vi "Main.vi"() -> ()   [LabVIEW 2017, in "MQTT.lvlib"]
doc: "This template is based from the Queued Message Handler design pattern and the Queued Message Handler Project Template that ships with LabVIEW 2014.\n\nThe main difference is that the Queue is private to this module and communication between modules is done via Broadcast and Requests events.\n\nRequests events are wrapped via public API methods and are handled in the Event handler loop in this VI.\nAny module can register for Broadcast events sent by this module.\n\nThe Event Handling Loop generates messages based on user interface actions.\n\nThe Message Handling Loop processes messages generated by the Event Handling Loop, or by other messages. The messages are string values, so new messages can be added easily to the Message Cases case structure in the Message Handling Loop. Each message cluster can also provide an optional value for Message Data, which is a variant that can be converted to whatever message-specific data is required.\n_____\nBased on Delacor QMH Project Template 3.1.0.34."
uses:
  MQTT.lvlib
  <vilib>/Delacor/Delacor QMH/Libraries/Cloneable Module Admin_class/Delacor_lib_QMH_Cloneable Module Admin.lvclass
  C:/Program Files (x86)/National Instruments/LabVIEW 2017/vi.lib/Delacor/Delacor QMH/Libraries/Module Admin_class/Delacor_lib_QMH_Module Admin.lvclass
  MessageTypedef.ctl
  Module Data--cluster.ctl
  OOP/MQTTclient.lvclass
  OOP/Dict/DICT.lvclass
  <vilib>/Delacor/Delacor QMH/Libraries/Message Queue_class/Delacor_lib_QMH_Message Queue.lvclass/Delacor_lib_QMH_Message Queue.ctl
  <vilib>/Delacor/Delacor QMH/Libraries/Cloneable Module Admin_class/Delacor_lib_QMH_Cloneable Module Admin.lvclass/Delacor_lib_QMH_Cloneable Module Admin.ctl
  Stop Argument--cluster.ctl
  <vilib>/Delacor/Delacor QMH/Libraries/Module Admin_class/Delacor_lib_QMH_Module Admin.lvclass/Delacor_lib_QMH_Module Admin.ctl
  Configure Argument--cluster.ctl
  Connect Argument--cluster.ctl
  disconnect Argument--cluster.ctl
  Subscrie Argument--cluster.ctl
  unsubscribe Argument--cluster.ctl
  Publish Argument--cluster.ctl
  broadcastTopic Argument--cluster.ctl
  PublishByAlias Argument--cluster.ctl
  addTopicAlias Argument--cluster.ctl
  <vilib>/Utility/miscctls.llb/LVPointTypeDef.ctl
  OOP/MQTT1/MQTT1.lvclass
  C:/Users/radzi01m/OneDrive - SIEMENSGAMESA/ISYS/MQTTGateway/OOP/MQTTclient.lvclass
  <vilib>/Delacor/Delacor QMH/Libraries/Message Queue_class/Delacor_lib_QMH_Enqueue Message (Single).vi
  <vilib>/Delacor/Delacor QMH/Libraries/Cloneable Module Admin_class/Delacor_lib_QMH_Get Module ID.vi
  <vilib>/Delacor/Delacor QMH/Libraries/Module Admin_class/Delacor_lib_QMH_Get External Launch.vi
  <vilib>/Utility/error.llb/Error Cluster From Error Code.vi
  <vilib>/ErrorRing/Error Ring.xnode
  <vilib>/Delacor/Delacor QMH/Libraries/Message Queue_class/Delacor_lib_QMH_Message Queue.lvclass
  Clone Registration/Clone Registration.lvlib
panel:
  in  "Simulate MHL Error":bool
  in  "Simulate EHL Error":bool
  out "error out":errorcluster
  in  "Module Admin":refnum<class "Delacor_lib_QMH_Cloneable Module Admin.lvclass">
  out "Status":string
  # "Other QMH Modules communicate with this Module via its Public API (wrappers for its Request Events).\n\nThis Module communicates with other Modules via its Broadcast Events.\nAny module that wants to get these messages, just registers for this module's Broadcast events."
  # "This template is for the Delacor Modified Queued Message Handler design pattern.\n\nSee the block diagram for more information on how to use this template."
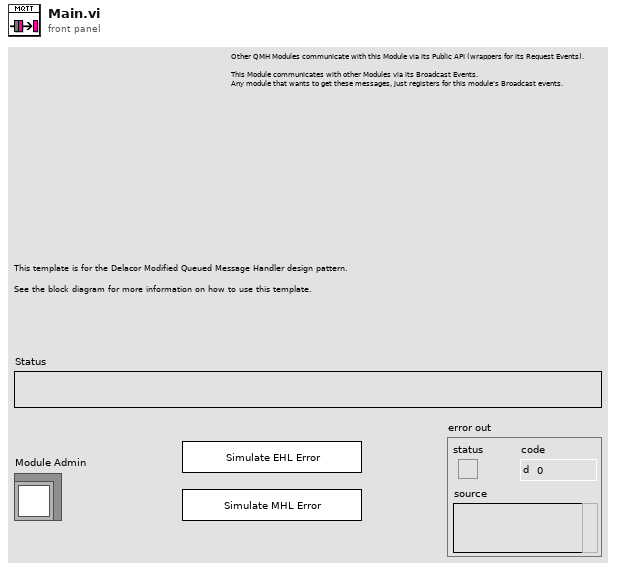
[diagram p1: front panel]
types:
  T1 = typedef "MQTT.lvlib/Request Events--cluster.ctl" = cluster{"Stop Module":refnum<user-event>, "Show Panel":refnum<user-event>, "Hide Panel":refnum<user-event>, "Show Diagram":refnum<user-event>, "Get Module Execution Status":refnum<user-event>, "Configure":refnum<user-event>, "Connect":refnum<user-event>, "disconnect":refnum<user-event>, "Subscrie":refnum<user-event>, "unsubscribe":refnum<user-event>, "Publish":refnum<user-event>, "Register Event":refnum<user-event>, "broadcastTopic":refnum<user-event>, "PublishByAlias":refnum<user-event>, "addTopicAlias":refnum<user-event>}
  T2 = typedef "MQTT.lvlib/Module Data--cluster.ctl" = cluster{"Status":string, "MQTTclient":refnum<class "MQTTclient.lvclass">, "DICT":refnum<class "DICT.lvclass">}
  T3 = typedef "MQTT.lvlib/Stop Argument--cluster.ctl" = cluster{"Origin":string, "Module ID":i32, "Exit via Stop Module Req?":bool, "Wait for Module to stop?":bool}
  T4 = typedef "MQTT.lvlib/Configure Argument--cluster.ctl" = cluster{"Module ID":i32, "JSON config":string}
  T5 = typedef "MQTT.lvlib/Connect Argument--cluster.ctl" = cluster{"Module ID":i32, "Boolean":bool}
  T6 = typedef "MQTT.lvlib/disconnect Argument--cluster.ctl" = cluster{"Module ID":i32, "Boolean":bool}
  T7 = typedef "MQTT.lvlib/Subscrie Argument--cluster.ctl" = cluster{"Module ID":i32, "Topic":string, "Alias":string}
  T8 = typedef "MQTT.lvlib/unsubscribe Argument--cluster.ctl" = cluster{"Module ID":i32, "Topic":string}
  T9 = typedef "MQTT.lvlib/Publish Argument--cluster.ctl" = cluster{"Module ID":i32, "Topic":string, "Payload":string}
  T10 = typedef "MQTT.lvlib/broadcastTopic Argument--cluster.ctl" = cluster{"Module ID":i32, "Topic":string, "Message":string}
  T11 = typedef "MQTT.lvlib/PublishByAlias Argument--cluster.ctl" = cluster{"Module ID":i32, "Alias":string, "Payload":string}
  T12 = typedef "MQTT.lvlib/addTopicAlias Argument--cluster.ctl" = cluster{"Module ID":i32, "Topic":string, "Alias":string}
  T13 = typedef "LVPointTypeDef.ctl" = cluster{"Horizontal":i16, "Vertical":i16}
  T14 = enum32{"Invalid", "Standard", "Closed", "Hidden", "Minimized", "Maximized"}
  T15 = enum32{"invalid lock state", "Not Locked", "Locked (No Password)", "Password-protected"}
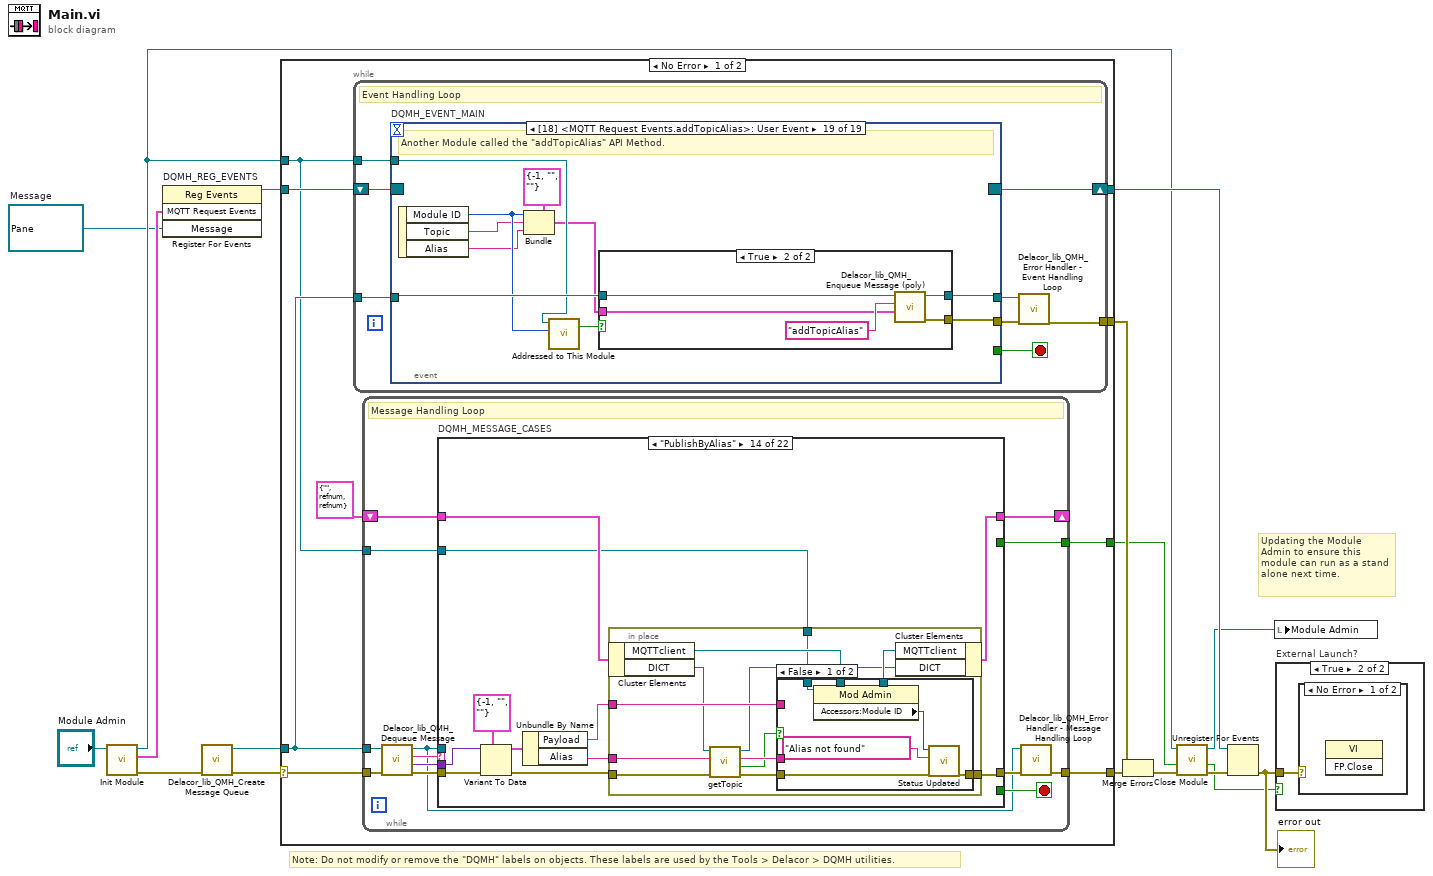
[diagram p0: block diagram]
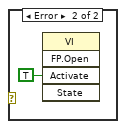
[diagram p3: hidden frame]
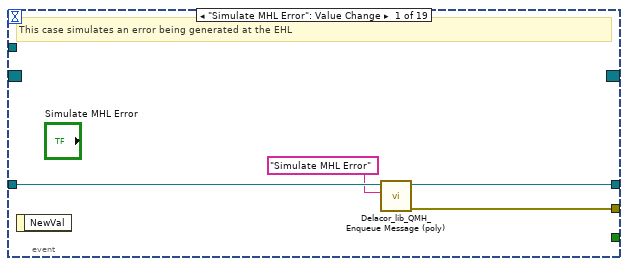
[diagram p4: hidden frame]
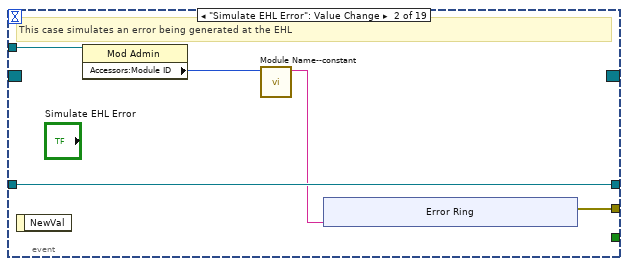
[diagram p5: hidden frame]
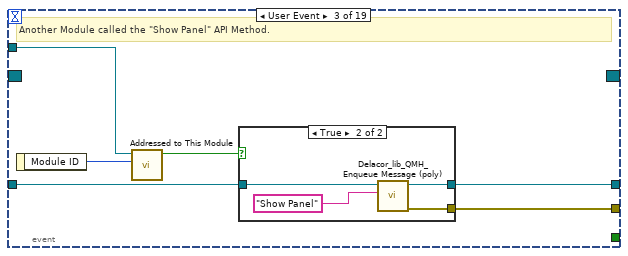
[diagram p6: hidden frame]
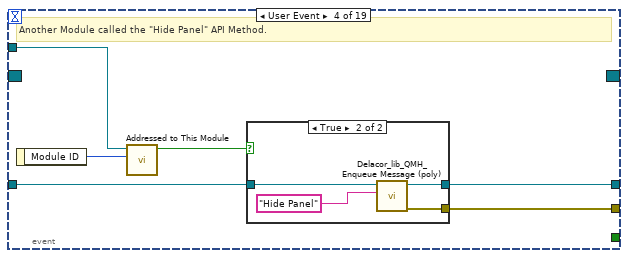
[diagram p8: hidden frame]
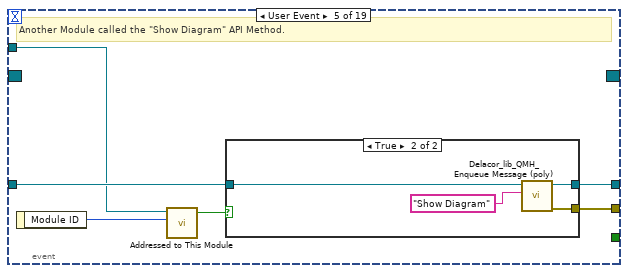
[diagram p10: hidden frame]
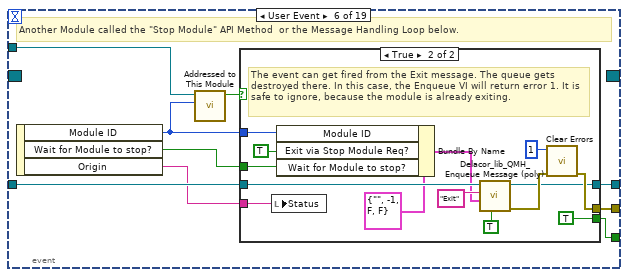
[diagram p12: hidden frame]
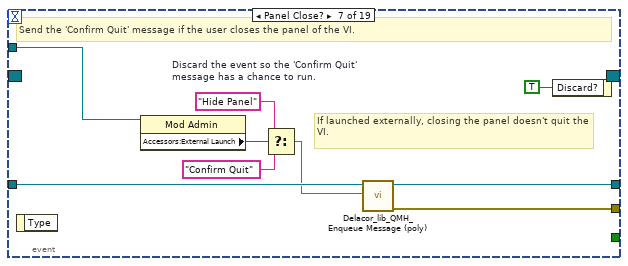
[diagram p14: hidden frame]
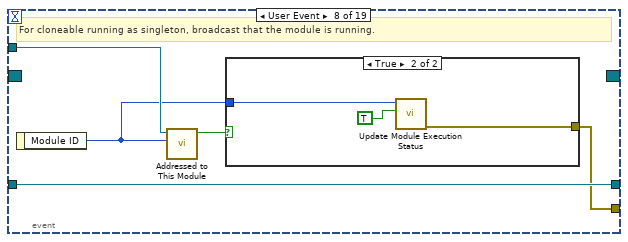
[diagram p15: hidden frame]
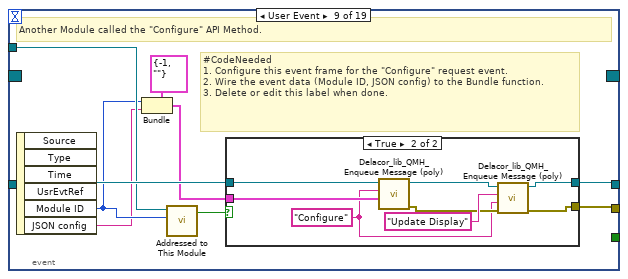
[diagram p17: hidden frame]
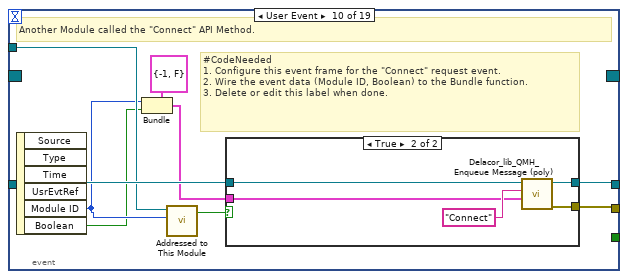
[diagram p19: hidden frame]
diagram:
  w1 = refnum<user-event> refnum  # Message
  # "Note: Do not modify or remove the \"DQMH\" labels on objects. These labels are used by the Tools > Delacor > DQMH utilities."
  # "Updating the Module Admin to ensure this module can run as a stand alone next time."
  n1 = call "Init Module.vi"("Cloneable Module Admin in"="Module Admin") -> ("error out"=w14:errorcluster, "MQTT Request Events"=w11:T1, "Cloneable Module Admin out"=w7:refnum<class "Delacor_lib_QMH_Cloneable Module Admin.lvclass">)  [unwired: 8 in]
  n2 = register-events "DQMH_REG_EVENTS"(w11, w1) -> (reference out=w12:refnum<event-registration>)  [unwired: 2 in, 1 out]
  n3 = call <vilib>:"Delacor_lib_QMH_Create Message Queue.vi"("error in (no error)"=w14) -> ("error out"=w2:errorcluster, "Message Queue"=w10:refnum<class "Delacor_lib_QMH_Message Queue.lvclass">)  [unwired: 9 in]
  n4 = case shown="No Error" w2 {
    selector: w2 -> [w20 w672]
    tunnel: [w26 w672] -> w15
    tunnel: [w25 w673] -> w13
    tunnel: w12 -> [w23 w673]
    tunnel: w10 -> [w22 _]
    tunnel: [w21 _] -> w16
    tunnel: w7 -> [w19 w668]
    tunnel: [w18 _] -> w5
    frame No Error {
      n5 = while {
        tunnel: w22 -> [w34]
        shift-right: [w27] -> w25
        shift-left: w23 -> [w33]
        tunnel: [w29] -> w21
        tunnel: w19 -> [w28]
        stop <- w31 stop-if-true
        # "Event Handling Loop"
        n6 = event "DQMH_EVENT_MAIN" shown="[18] <MQTT Request Events.addTopicAlias>: User Event" {
          selector: w33 -> [_ _ _ _ _ _ _ _ _ _ w159 _ _ _ w227 _ _ _ _]
          dyn-events: [_ _ _ _ _ _ _ _ _ _ w158 _ _ _ w226 _ _ _ _] -> w27
          timeout: _ -> [_ _ _ _ _ _ _ _ _ _ _ _ _ _ _ _ _ _ _]
          tunnel: [_ _ _ _ _ w87 _ _ _ _ _ _ _ _ _ _ _ _ _] -> w31
          tunnel: w34 -> [w38 w43 w56 w67 w78 w90 w115 w119 w133 w151 w167 w187 w202 w218 w232 w244 w254 w270 w286]
          tunnel: [w36 w42 w54 w65 w74 w92 w114 w118 w127 w145 w161 w181 w196 w212 _ w242 w245 w261 w277] -> w32
          tunnel: [w37 w43 w55 w66 w77 w91 w113 w119 w132 w150 w166 w186 w201 w217 w231 w244 w253 w269 w285] -> w30
          tunnel: w28 -> [_ w41 w51 w62 w75 w89 w109 w120 w130 w148 w164 w184 w199 w215 w229 w243 w251 w267 w283]
          event "Simulate MHL Error": Value Change {
            # "This case simulates an error being generated at the EHL"
            n7 = event-data() -> ()  [unwired: 1 in, 1 out]
            n8 = call-poly <vilib>:"Delacor_lib_QMH_Enqueue Message (poly).vi"("Message"="Simulate MHL Error", "Message Queue in"=w38) -> ("error out"=w36:errorcluster, "Message Queue out"=w37:refnum<class "Delacor_lib_QMH_Message Queue.lvclass">)  [unwired: 8 in]
          }
          event "Simulate EHL Error": Value Change {
            # "This case simulates an error being generated at the EHL"
            n9 = event-data() -> ()  [unwired: 1 in, 1 out]
            n10 = property class="Mod Admin"(reference=w41) -> ("Accessors:Module ID"=w40:i32)  [unwired: 1 in, 2 out]
            n11 = call "Module Name--constant.vi"("Module ID"=w40) -> ("Module Name"=w39:string)  [unwired: 10 in]
            n12 = xnode "Error Ring"("parameter 0"=w39) -> ("error out"=w42:errorcluster)
          }
          event User Event {
            # "Another Module called the \"Show Panel\" API Method."
            n13 = event-data() -> ("Module ID"=w53:i32)  [unwired: 1 in]
            n14 = call "Addressed to This Module.vi"("Module ID from Argument"=w53, "Module Admin"=w51) -> ("Addressed to this instance?"=w52:bool)  [unwired: 8 in, 1 out]
            n15 = case shown="True" w52 {
              tunnel: w56 -> [w57 w61]
              tunnel: [w57 w60] -> w55
              tunnel: [_ w59] -> w54
              frame False {
              }
              frame True {
                n16 = call-poly <vilib>:"Delacor_lib_QMH_Enqueue Message (poly).vi"("Message"="Show Panel", "Message Queue in"=w61) -> ("error out"=w59:errorcluster, "Message Queue out"=w60:refnum<class "Delacor_lib_QMH_Message Queue.lvclass">)  [unwired: 8 in]
              }
            }
          }
          event User Event {
            # "Another Module called the \"Hide Panel\" API Method."
            n17 = event-data() -> ("Module ID"=w64:i32)  [unwired: 1 in]
            n18 = call "Addressed to This Module.vi"("Module ID from Argument"=w64, "Module Admin"=w62) -> ("Addressed to this instance?"=w63:bool)  [unwired: 8 in, 1 out]
            n19 = case shown="True" w63 {
              tunnel: w67 -> [w68 w72]
              tunnel: [w68 w71] -> w66
              tunnel: [_ w70] -> w65
              frame False {
              }
              frame True {
                n20 = call-poly <vilib>:"Delacor_lib_QMH_Enqueue Message (poly).vi"("Message"="Hide Panel", "Message Queue in"=w72) -> ("error out"=w70:errorcluster, "Message Queue out"=w71:refnum<class "Delacor_lib_QMH_Message Queue.lvclass">)  [unwired: 8 in]
              }
            }
          }
          event User Event {
            # "Another Module called the \"Show Diagram\" API Method."
            n21 = event-data() -> ("Module ID"=w73:i32)  [unwired: 1 in]
            n22 = call "Addressed to This Module.vi"("Module ID from Argument"=w73, "Module Admin"=w75) -> ("Addressed to this instance?"=w76:bool)  [unwired: 8 in, 1 out]
            n23 = case shown="True" w76 {
              tunnel: w78 -> [w79 w83]
              tunnel: [w79 w82] -> w77
              tunnel: [_ w80] -> w74
              frame False {
              }
              frame True {
                n24 = call-poly <vilib>:"Delacor_lib_QMH_Enqueue Message (poly).vi"("Message"="Show Diagram", "Message Queue in"=w83) -> ("error out"=w80:errorcluster, "Message Queue out"=w82:refnum<class "Delacor_lib_QMH_Message Queue.lvclass">)  [unwired: 8 in]
              }
            }
          }
          event User Event {
            # "Another Module called the \"Stop Module\" API Method  or the Message Handling Loop below."
            n25 = event-data() -> ("Module ID"=w85:i32, "Wait for Module to stop?"=w86:bool, "Origin"=w84:string)  [unwired: 1 in]
            n26 = call "Addressed to This Module.vi"("Module ID from Argument"=w85, "Module Admin"=w89) -> ("Addressed to this instance?"=w88:bool)  [unwired: 8 in, 1 out]
            n27 = case shown="True" w88 {
              tunnel: [_ w103] -> w92
              tunnel: [w93 w102] -> w91
              tunnel: w90 -> [w93 w101]
              tunnel: [_ TRUE] -> w87
              tunnel: w86 -> [_ w96]
              tunnel: w85 -> [_ w98]
              tunnel: w84 -> [_ w94]
              frame False {
              }
              frame True {
                # "The event can get fired from the Exit message. The queue gets destroyed there. In this case, the Enqueue VI will return error 1. It is safe to ignore, because the module is already exiting."
                n28 = local write "Status"(w94) -> ()
                n29 = Bundle By Name(cluster=T3 {"Origin"="", "Module ID"=-1, "Exit via Stop Module Req?"=FALSE, "Wait for Module to stop?"=FALSE} ("Stop Argument"), "Module ID"=w98, "Exit via Stop Module Req?"=TRUE, "Wait for Module to stop?"=w96) -> (w95:T3)
                n30 = call-poly <vilib>:"Delacor_lib_QMH_Enqueue Message (poly).vi"("Priority Message? (F)"=TRUE, "Message Data"=w95, "Message"="Exit", "Message Queue in"=w101) -> ("error out"=w106:errorcluster, "Message Queue out"=w102:refnum<class "Delacor_lib_QMH_Message Queue.lvclass">)  [unwired: 6 in]
                n31 = call <vilib>:"Clear Errors.vi"("error in (no error)"=w106, "specific error code to clear (0: all)"=1) -> ("error out"=w103:errorcluster)  [unwired: 4 in, 1 out]
              }
            }
          }
          event Panel Close? {
            w116 = TRUE  # Discard the event so the 'Confirm Quit' message has a chance to run.
            # "If launched externally, closing the panel doesn't quit the VI."
            # "Send the 'Confirm Quit' message if the user closes the panel of the VI."
            n32 = event-data() -> ()  [unwired: 1 in, 1 out]
            n33 = property class="Mod Admin"(reference=w109) -> ("Accessors:External Launch"=w108:bool)  [unwired: 1 in, 2 out]
            n34 = Select(t="Hide Panel" ("Message"), s=w108, f="Confirm Quit" ("Message")) -> (s? t:f=w110:string)
            n35 = call-poly <vilib>:"Delacor_lib_QMH_Enqueue Message (poly).vi"("Message"=w110, "Message Queue in"=w115) -> ("error out"=w114:errorcluster, "Message Queue out"=w113:refnum<class "Delacor_lib_QMH_Message Queue.lvclass">)  [unwired: 8 in]
            n36 = event-data("Discard?"=w116) -> ()  [unwired: 1 in, 1 out]
          }
          event User Event {
            # "For cloneable running as singleton, broadcast that the module is running."
            n37 = event-data() -> ("Module ID"=w117:i32)  [unwired: 1 in]
            n38 = call "Addressed to This Module.vi"("Module ID from Argument"=w117, "Module Admin"=w120) -> ("Addressed to this instance?"=w121:bool)  [unwired: 8 in, 1 out]
            n39 = case shown="True" w121 {
              tunnel: [_ w124] -> w118
              tunnel: w117 -> [_ w123]
              frame False {
              }
              frame True {
                n40 = call "Update Module Execution Status.vi"("Running?"=TRUE, "Module ID"=w123) -> ("error out"=w124:errorcluster)  [unwired: 9 in]
              }
            }
          }
          event User Event {
            # "#CodeNeeded\n1. Configure this event frame for the \"Configure\" request event.\n2. Wire the event data (Module ID, JSON config) to the Bundle function.\n3. Delete or edit this label when done."
            # "Another Module called the \"Configure\" API Method."
            n41 = event-data() -> ("Module ID"=w126:i32, "JSON config"=w125:string)  [unwired: 1 in, 4 out]
            n42 = Bundle(cluster=T4 {"Module ID"=-1, "JSON config"=""} ("Configure Argument"), "Module ID"=w126, "JSON config"=w125) -> (w128:T4)
            n43 = call "Addressed to This Module.vi"("Module ID from Argument"=w126, "Module Admin"=w130) -> ("Addressed to this instance?"=w131:bool)  [unwired: 8 in, 1 out]
            n44 = case shown="True" w131 {
              tunnel: w133 -> [w134 w142]
              tunnel: [w134 w138] -> w132
              tunnel: w128 -> [_ w141]
              tunnel: [_ w137] -> w127
              frame False {
              }
              frame True {
                w135 = "Configure"
                n45 = call-poly <vilib>:"Delacor_lib_QMH_Enqueue Message (poly).vi"("Message Data"=w141, "Message"=w135, "Message Queue in"=w142) -> ("error out"=w136:errorcluster, "Message Queue out"=w139:refnum<class "Delacor_lib_QMH_Message Queue.lvclass">)  [unwired: 7 in]
                n46 = call-poly <vilib>:"Delacor_lib_QMH_Enqueue Message (poly).vi"("error in (no error)"=w136, "Message Data"=w135, "Message"="Update Display", "Message Queue in"=w139) -> ("error out"=w137:errorcluster, "Message Queue out"=w138:refnum<class "Delacor_lib_QMH_Message Queue.lvclass">)  [unwired: 6 in]
              }
            }
          }
          event User Event {
            # "#CodeNeeded\n1. Configure this event frame for the \"Connect\" request event.\n2. Wire the event data (Module ID, Boolean) to the Bundle function.\n3. Delete or edit this label when done."
            # "Another Module called the \"Connect\" API Method."
            n47 = event-data() -> ("Module ID"=w144:i32, "Boolean"=w143:bool)  [unwired: 1 in, 4 out]
            n48 = Bundle(cluster=T5 {"Module ID"=-1, "Boolean"=FALSE} ("Connect Argument"), "Module ID"=w144, "Boolean"=w143) -> (w146:T5)
            n49 = call "Addressed to This Module.vi"("Module ID from Argument"=w144, "Module Admin"=w148) -> ("Addressed to this instance?"=w149:bool)  [unwired: 8 in, 1 out]
            n50 = case shown="True" w149 {
              tunnel: w151 -> [w152 w157]
              tunnel: [w152 w156] -> w150
              tunnel: w146 -> [_ w154]
              tunnel: [_ w153] -> w145
              frame False {
              }
              frame True {
                n51 = call-poly <vilib>:"Delacor_lib_QMH_Enqueue Message (poly).vi"("Message Data"=w154, "Message"="Connect", "Message Queue in"=w157) -> ("error out"=w153:errorcluster, "Message Queue out"=w156:refnum<class "Delacor_lib_QMH_Message Queue.lvclass">)  [unwired: 7 in]
              }
            }
          }
          event User Event {
            # "Another Module called the \"disconnect\" API Method."
            n52 = event-data() -> ("Module ID"=w160:i32)  [unwired: 1 in, 5 out]
            n53 = Bundle(cluster=T6 {"Module ID"=-1, "Boolean"=FALSE} ("disconnect Argument"), "Module ID"=w160) -> (w162:T6)  [unwired: 1 in]
            n54 = call "Addressed to This Module.vi"("Module ID from Argument"=w160, "Module Admin"=w164) -> ("Addressed to this instance?"=w165:bool)  [unwired: 8 in, 1 out]
            n55 = case shown="True" w165 {
              tunnel: w167 -> [w169 w177]
              tunnel: [w169 w176] -> w166
              tunnel: w162 -> [_ w174]
              tunnel: [_ w173] -> w161
              tunnel: w159 -> [w168 w172]
              tunnel: [w168 w171] -> w158
              frame False {
              }
              frame True {
                w170 = refnum<user-event> refnum  # Message
                n56 = register-events "DQMH_REG_EVENTS"(reference=w172, w170) -> (reference out=w171:refnum<event-registration>)  [unwired: 2 in, 1 out]
                n57 = call-poly <vilib>:"Delacor_lib_QMH_Enqueue Message (poly).vi"("Message Data"=w174, "Message"="disconnect", "Message Queue in"=w177) -> ("error out"=w173:errorcluster, "Message Queue out"=w176:refnum<class "Delacor_lib_QMH_Message Queue.lvclass">)  [unwired: 7 in]
              }
            }
          }
          event User Event {
            # "Another Module called the \"Subscrie\" API Method."
            n58 = event-data() -> ("Module ID"=w179:i32, "Topic"=w180:string, "Alias"=w178:string)  [unwired: 1 in, 4 out]
            n59 = Bundle(cluster=T7 {"Module ID"=-1, "Topic"="", "Alias"=""} ("Subscrie Argument"), "Module ID"=w179, "Topic"=w180, "Alias"=w178) -> (w182:T7)
            n60 = call "Addressed to This Module.vi"("Module ID from Argument"=w179, "Module Admin"=w184) -> ("Addressed to this instance?"=w185:bool)  [unwired: 8 in, 1 out]
            n61 = case shown="True" w185 {
              tunnel: w187 -> [w188 w193]
              tunnel: [w188 w192] -> w186
              tunnel: w182 -> [_ w190]
              tunnel: [_ w189] -> w181
              frame False {
              }
              frame True {
                n62 = call-poly <vilib>:"Delacor_lib_QMH_Enqueue Message (poly).vi"("Message Data"=w190, "Message"="Subscrie", "Message Queue in"=w193) -> ("error out"=w189:errorcluster, "Message Queue out"=w192:refnum<class "Delacor_lib_QMH_Message Queue.lvclass">)  [unwired: 7 in]
              }
            }
          }
          event User Event {
            # "#CodeNeeded\n1. Configure this event frame for the \"unsubscribe\" request event.\n2. Wire the event data (Module ID, Topic) to the Bundle function.\n3. Delete or edit this label when done."
            # "Another Module called the \"unsubscribe\" API Method."
            n63 = event-data() -> ("Module ID"=w194:i32, "Topic"=w195:string)  [unwired: 1 in, 4 out]
            n64 = Bundle(cluster=T8 {"Module ID"=-1, "Topic"=""} ("unsubscribe Argument"), "Module ID"=w194, "Topic"=w195) -> (w197:T8)
            n65 = call "Addressed to This Module.vi"("Module ID from Argument"=w194, "Module Admin"=w199) -> ("Addressed to this instance?"=w200:bool)  [unwired: 8 in, 1 out]
            n66 = case shown="True" w200 {
              tunnel: w202 -> [w203 w208]
              tunnel: [w203 w207] -> w201
              tunnel: w197 -> [_ w205]
              tunnel: [_ w204] -> w196
              frame False {
              }
              frame True {
                n67 = call-poly <vilib>:"Delacor_lib_QMH_Enqueue Message (poly).vi"("Message Data"=w205, "Message"="unsubscribe", "Message Queue in"=w208) -> ("error out"=w204:errorcluster, "Message Queue out"=w207:refnum<class "Delacor_lib_QMH_Message Queue.lvclass">)  [unwired: 7 in]
              }
            }
          }
          event User Event {
            # "#CodeNeeded\n1. Configure this event frame for the \"Publish\" request event.\n2. Wire the event data (Module ID, Boolean) to the Bundle function.\n3. Delete or edit this label when done."
            # "Another Module called the \"Publish\" API Method."
            n68 = event-data() -> ("Module ID"=w211:i32, "Topic"=w210:string, "Payload"=w209:string)  [unwired: 1 in, 4 out]
            n69 = Bundle(cluster=T9 {"Module ID"=-1, "Topic"="", "Payload"=""} ("Publish Argument"), "Module ID"=w211, "Topic"=w210, "Payload"=w209) -> (w213:T9)
            n70 = call "Addressed to This Module.vi"("Module ID from Argument"=w211, "Module Admin"=w215) -> ("Addressed to this instance?"=w216:bool)  [unwired: 8 in, 1 out]
            n71 = case shown="True" w216 {
              tunnel: w218 -> [w219 w224]
              tunnel: [w219 w223] -> w217
              tunnel: w213 -> [_ w221]
              tunnel: [_ w220] -> w212
              frame False {
              }
              frame True {
                n72 = call-poly <vilib>:"Delacor_lib_QMH_Enqueue Message (poly).vi"("Message Data"=w221, "Message"="Publish", "Message Queue in"=w224) -> ("error out"=w220:errorcluster, "Message Queue out"=w223:refnum<class "Delacor_lib_QMH_Message Queue.lvclass">)  [unwired: 7 in]
              }
            }
          }
          event User Event {
            # "Another Module called the \"Register Event\" API Method."
            n73 = event-data() -> ("Module ID"=w228:i32, "Message Received"=w225:refnum<user-event>)  [unwired: 1 in, 4 out]
            n74 = call "Addressed to This Module.vi"("Module ID from Argument"=w228, "Module Admin"=w229) -> ("Addressed to this instance?"=w230:bool)  [unwired: 8 in, 1 out]
            n75 = case shown="True" w230 {
              tunnel: w232 -> [w234 w238]
              tunnel: [w234 w238] -> w231
              tunnel: w227 -> [w233 w237]
              tunnel: [w233 w236] -> w226
              tunnel: w225 -> [_ w235]
              frame False {
              }
              frame True {
                n76 = register-events(reference=w237, w235) -> (reference out=w236:refnum<event-registration>)  [unwired: 2 in, 1 out]
              }
            }
          }
          event User Event {
            n77 = event-data() -> ("Topic"=w240:string, "Payload"=w239:string)  [unwired: 1 in, 4 out]
            n78 = property class="Mod Admin"(reference=w243) -> ("Accessors:Module ID"=w241:i32)  [unwired: 1 in, 2 out]
            n79 = call "broadcastTopic.vi"("Message"=w239, "Topic"=w240, "Module ID"=w241) -> ("error out"=w242:errorcluster)  [unwired: 8 in]
          }
          event User Event {
            # "Another Module called the \"broadcastTopic\" API Method."
            n80 = event-data() -> ("Module ID"=w248:i32, "Topic"=w247:string, "Message"=w246:string)  [unwired: 1 in]
            n81 = Bundle(cluster=T10 {"Module ID"=-1, "Topic"="", "Message"=""} ("broadcastTopic Argument"), "Module ID"=w248, "Topic"=w247, "Message"=w246) -> (w249:T10)
            n82 = call "Addressed to This Module.vi"("Module ID from Argument"=w248, "Module Admin"=w251) -> ("Addressed to this instance?"=w252:bool)  [unwired: 8 in, 1 out]
            n83 = case shown="True" w252 {
              tunnel: w254 -> [w255 w260]
              tunnel: [w255 w259] -> w253
              tunnel: w249 -> [_ w257]
              tunnel: [_ w256] -> w245
              frame False {
              }
              frame True {
                n84 = call-poly <vilib>:"Delacor_lib_QMH_Enqueue Message (poly).vi"("Message Data"=w257, "Message"="broadcastTopic", "Message Queue in"=w260) -> ("error out"=w256:errorcluster, "Message Queue out"=w259:refnum<class "Delacor_lib_QMH_Message Queue.lvclass">)  [unwired: 7 in]
              }
            }
          }
          event User Event {
            # "Another Module called the \"PublishByAlias\" API Method."
            n85 = event-data() -> ("Module ID"=w264:i32, "Alias"=w263:string, "Payload"=w262:string)  [unwired: 1 in]
            n86 = Bundle(cluster=T11 {"Module ID"=-1, "Alias"="", "Payload"=""} ("PublishByAlias Argument"), "Module ID"=w264, "Alias"=w263, "Payload"=w262) -> (w265:T11)
            n87 = call "Addressed to This Module.vi"("Module ID from Argument"=w264, "Module Admin"=w267) -> ("Addressed to this instance?"=w268:bool)  [unwired: 8 in, 1 out]
            n88 = case shown="True" w268 {
              tunnel: w270 -> [w271 w276]
              tunnel: [w271 w275] -> w269
              tunnel: w265 -> [_ w273]
              tunnel: [_ w272] -> w261
              frame False {
              }
              frame True {
                n89 = call-poly <vilib>:"Delacor_lib_QMH_Enqueue Message (poly).vi"("Message Data"=w273, "Message"="PublishByAlias", "Message Queue in"=w276) -> ("error out"=w272:errorcluster, "Message Queue out"=w275:refnum<class "Delacor_lib_QMH_Message Queue.lvclass">)  [unwired: 7 in]
              }
            }
          }
          event User Event {
            # "Another Module called the \"addTopicAlias\" API Method."
            n90 = event-data() -> ("Module ID"=w280:i32, "Topic"=w279:string, "Alias"=w278:string)  [unwired: 1 in]
            n91 = Bundle(cluster=T12 {"Module ID"=-1, "Topic"="", "Alias"=""} ("addTopicAlias Argument"), "Module ID"=w280, "Topic"=w279, "Alias"=w278) -> (w281:T12)
            n92 = call "Addressed to This Module.vi"("Module ID from Argument"=w280, "Module Admin"=w283) -> ("Addressed to this instance?"=w284:bool)  [unwired: 8 in, 1 out]
            n93 = case shown="True" w284 {
              tunnel: w286 -> [w287 w292]
              tunnel: [w287 w291] -> w285
              tunnel: w281 -> [_ w289]
              tunnel: [_ w288] -> w277
              frame False {
              }
              frame True {
                n94 = call-poly <vilib>:"Delacor_lib_QMH_Enqueue Message (poly).vi"("Message Data"=w289, "Message"="addTopicAlias", "Message Queue in"=w292) -> ("error out"=w288:errorcluster, "Message Queue out"=w291:refnum<class "Delacor_lib_QMH_Message Queue.lvclass">)  [unwired: 7 in]
              }
            }
          }
        }
        n95 = call-dynamic "Delacor_lib_QMH_Error Handler - Event Handling Loop.vi"("error in (no error)"=w32, "Message Queue in"=w30) -> ("dup error in"=w29:errorcluster)  [unwired: 8 in, 1 out]
      }
      n96 = while {
        tunnel: w22 -> [w297]
        shift-right: [w303] -> _
        shift-left: T2 {"Status"="", "MQTTclient"=refnum, "DICT"=refnum} ("Data Cluster") -> [w304]
        tunnel: w20 -> [w301]
        tunnel: [w295] -> w26
        tunnel: w19 -> [w294]
        tunnel: [w293] -> w18
        stop <- w302 stop-if-true
        # "Message Handling Loop"
        n97 = call-dynamic "Delacor_lib_QMH_Dequeue Message.vi"("error in (no error)"=w301, "Message Queue in"=w297) -> ("error out"=w300:errorcluster, "Message Data"=w298:variant, "Message"=w299:string, "Message Queue out"=w296:refnum<class "Delacor_lib_QMH_Message Queue.lvclass">)  [unwired: 6 in]
        n98 = case "DQMH_MESSAGE_CASES" shown="\"PublishByAlias\"" w299 {
          selector: w299 -> [_ _ _ _ _ _ _ _ _ _ _ _ _ _ _ _ _ _ _ _ _ w655]
          tunnel: w296 -> [_ _ _ _ _ _ _ _ _ _ _ _ _ _ _ _ _ w595 _ w628 w649 _]
          tunnel: w300 -> [w322 w338 w346 w352 w355 w376 w385 w399 w420 w434 w452 w468 w503 w525 w566 w590 w593 w604 w617 w627 w651 _]
          tunnel: [w316 w339 w346 w352 w354 w374 w378 w392 w415 w429 w447 w464 w499 w520 w553 w588 w591 w594 w615 w626 w646 w656] -> w305
          tunnel: w304 -> [w321 w340 w345 w351 w356 w375 w381 w395 w417 w427 w445 w463 w494 w517 w561 w589 w592 w603 w616 w631 w633 w657]
          tunnel: [w306 w340 w345 w351 w356 w375 w380 w394 w416 w426 w444 w462 w493 w516 w560 w589 w592 w603 w616 w631 w633 w657] -> w303
          tunnel: [_ _ _ _ _ _ _ _ _ _ _ _ _ _ _ _ _ _ _ _ w648 _] -> w302
          tunnel: w298 -> [_ w337 _ _ _ _ w384 w398 w419 w433 w451 w467 w502 w524 w565 _ _ w602 _ _ w642 _]
          tunnel: w294 -> [w313 w332 w343 w350 w353 _ _ _ _ _ _ w458 _ w515 w552 _ _ w599 w612 _ w638 w653]
          tunnel: [_ _ _ _ _ _ _ _ _ _ _ _ _ _ _ _ _ _ _ _ w640 _] -> w293
          frame "Initialize" {
            w320 = "Initial Message" ("Initial Message")
            # "Initialize - Any operation that needs to be done before the module can receive messages. Synchronize Caller Events.vi will inform Start Module.vi that the module has launched and is ready to receive messages. Module Did Init.vi will broadcast that the module initialized."
            n99 = call "Synchronize Caller Events.vi"("error in (no error)"=w322, "Module Admin"=w313) -> ("error out"=w317:errorcluster, "Module Admin out"=w312:refnum<class "Delacor_lib_QMH_Cloneable Module Admin.lvclass">)  [unwired: 8 in]
            n100 = property class="Mod Admin"(reference=w312) -> ("Accessors:Module ID"=w315:i32, "Accessors:External Launch"=w314:bool)  [unwired: 1 in, 2 out]
            n101 = Bundle By Name(cluster=w321, "Status"=w320, "MQTTclient"=refnum<class "MQTT1.lvclass"> refnum ("MQTT1.lvclass")) -> (w308:T2)
            n102 = local write "Status"(w320) -> ()
            n103 = call "Module Name--constant.vi"("Module ID"=w315) -> ("Module Name"=w326:string)  [unwired: 10 in]
            n104 = Unbundle By Name(w308) -> ("DICT"=w309:refnum<class "DICT.lvclass">)
            n105 = call-dynamic "clear.vi"("DICT in"=w309) -> ("DICT out"=w307:refnum<class "DICT.lvclass">)  [unwired: 9 in, 1 out]
            n106 = property class="VI"("Front Panel.Title"=w326) -> (reference out=w329:refnum<vi>, error out=w330:errorcluster)  [unwired: 2 in]
            n107 = Bundle By Name(cluster=w308, "DICT"=w307) -> (w306:T2)
            n108 = Select(t=T14."Hidden" ("State"), s=w314, f=T14."Standard" ("State")) -> (s? t:f=w323:T14)
            n109 = invoke class="VI" method="FP.Open"(reference=w329, error in=w330, "State"=w323) -> (reference out=w328:refnum<vi>, error out=w327:errorcluster)  [unwired: 2 in, 3 out]
            n110 = call "Module Name--constant.vi"("Module ID"=w315) -> ("Module Name"=w318:string)  [unwired: 10 in]
            n111 = invoke class="VI" method="FP.Center"(reference=w328, error in=w327) -> ()  [unwired: 1 in, 3 out]
            n112 = property on="Pane" class="Pane"("Origin"=T13 {"Horizontal"=0, "Vertical"=0}) -> ()  [unwired: 2 in, 2 out]
            n113 = call "Module Did Init.vi"("error in (no error)"=w317, "Initialized?"=TRUE, "Origin"=w318, "Module ID"=w315) -> ("error out"=w316:errorcluster)  [unwired: 7 in]
          }
          frame "Update Display" {
            # "Broadcast updated status to any VI registered to listen to this module's broadcast events."
            # "Convert the message data to a string to display in the Status indicator."
            # "#CodeRecommended - If you wish to decouple the Message Handling Loop from your user interface, consider creating User Events (like the \"Stop\" event in this VI) to message the Event Handling Loop whenever the user interface needs updating."
            # "Update Display - Update user interface here."
            n114 = Variant To Data(error in=w338, type="", Variant=w337) -> (data=w335:string, error out=w334:errorcluster)
            "Status" <- w335
            n115 = property class="Mod Admin"(reference=w332) -> ("Accessors:Module ID"=w331:i32)  [unwired: 1 in, 2 out]
            n116 = call "Status Updated.vi"("error in (no error)"=w334, "Status"=w335, "Module ID"=w331) -> ("error out"=w333:errorcluster)  [unwired: 8 in]
            n117 = Merge Errors(w333) -> (w339:errorcluster)
          }
          frame "Show Panel" {
            # "Show the panel of this VI, and send a status updated message to let listeners know."
            n118 = property class="Mod Admin"(reference=w343) -> ("Accessors:Module ID"=w342:i32)  [unwired: 1 in, 2 out]
            n119 = call "Status Updated.vi"("Status"="Panel shown." ("format string"), "Module ID"=w342) -> ()  [unwired: 9 in, 1 out]
            n120 = invoke class="VI" method="FP.Open"("Activate"=TRUE ("Activate?")) -> ()  [unwired: 4 in, 5 out]
          }
          frame "Hide Panel" {
            # "Hide the panel of this VI, and send a status updated message to let listeners know."
            n121 = property class="Mod Admin"(reference=w350) -> ("Accessors:Module ID"=w349:i32)  [unwired: 1 in, 2 out]
            n122 = call "Status Updated.vi"("Status"="Panel hidden." ("format string"), "Module ID"=w349) -> ()  [unwired: 9 in, 1 out]
            n123 = invoke class="VI" method="FP.Open"("State"=T14."Hidden") -> ()  [unwired: 4 in, 5 out]
          }
          frame "Show Diagram" {
            # "Show Diagram - Show the block diagram of this VI. Used as a debugging tool. There is a button in the module tester that fires the Show Diagram request, which runs this message. Note that the diagram will not be displayed if it is password-protected and the password is not in the cache."
            n124 = disable-structure shown="RUN_TIME_ENGINE==False" {
              disable-tunnel: [w365 w373] -> w354
              disable-tunnel: w355 -> [w364 w373]
              disable-tunnel: w353 -> [w357 _]
              frame condition #0 (active) {
                # "functionality not available in exe"
                n125 = invoke class="VI" method="Lock State.Get"(error in=w364) -> (error out=w363:errorcluster, "Get Lock State"=w362:T15, "pwd in cache"=w359:bool)  [unwired: 3 in, 1 out]
                n126 = Equal?(x=T15."Password-protected", y=w362) -> (x = y?=w360:bool)
                n127 = Compound Arithmetic op=AND(w360, invert w359) -> (w358:bool)
                n128 = case shown="False" w358 {
                  tunnel: [w370 w372] -> w365
                  tunnel: w363 -> [w369 w372]
                  tunnel: w357 -> [w366 _]
                  frame False {
                    n129 = property class="Mod Admin"(reference=w366) -> ("Accessors:Module ID"=w367:i32)  [unwired: 1 in, 2 out]
                    n130 = property class="VI"(error in=w369, "BDWin.Open"=TRUE ("Block Diagram Window:Open")) -> (error out=w370:errorcluster)  [unwired: 1 in, 1 out]
                    n131 = call "Status Updated.vi"("Status"="Block Diagram shown." ("format string"), "Module ID"=w367) -> ()  [unwired: 9 in, 1 out]
                  }
                  frame True {
                    # "Password-protected VI, and the password is not in the cache. Do not show the diagram."
                  }
                }
              }
              frame condition #1 {
              }
            }
          }
          frame "--- Module Specific ---" {
            # "Separator -- The following cases handle messages specific to this Module."
            n132 = Merge Errors(w376) -> (w374:errorcluster)
          }
          frame "Configure" {
            # "Pass configuration  to module as JSON encoded string"
            n133 = Variant To Data(error in=w385, type=T4 {"Module ID"=-1, "JSON config"=""} ("Configure Argument"), Variant=w384) -> (data=w382:T4, error out=w379:errorcluster)
            n134 = Unbundle By Name(w382) -> ("JSON config"=w377:string)
            n135 = in-place {
              in-place-border: w379 -> [w388]
              in-place-border: [w387] -> w378
              in-place-border: w377 -> [w386]
              n136 = in-place-cluster #1(w381) -> ("MQTTclient"=w390:refnum<class "MQTTclient.lvclass">)
              n137 = call-dynamic "Config.vi"("error in (no error)"=w388, "JSON config"=w386, "MQTTclient in"=w390) -> ("error out"=w387:errorcluster, "MQTTclient out"=w389:refnum<class "MQTTclient.lvclass">)  [unwired: 7 in]
              n138 = in-place-cluster #1("MQTTclient"=w389) -> (w380:T2)
            }
          }
          frame "Connect" {
            n139 = Variant To Data(error in=w399, type=T5 {"Module ID"=-1, "Boolean"=FALSE} ("Connect Argument"), Variant=w398) -> (data=w396:T5, error out=w393:errorcluster)
            n140 = Unbundle By Name(w396) -> ("Module ID"=w391:i32)
            n141 = in-place {
              in-place-border: w393 -> [w412]
              in-place-border: [w405] -> w392
              in-place-border: w391 -> [w404]
              n142 = in-place-cluster #2(w395) -> ("MQTTclient"=w413:refnum<class "MQTTclient.lvclass">)
              n143 = call-dynamic "connect.vi"("error in (no error)"=w412, "MQTTclient in"=w413) -> ("error out"=w411:errorcluster, "Status"=w400:string, "Message"=w410:refnum<user-event>, "MQTTclient out"=w409:refnum<class "MQTTclient.lvclass">)  [unwired: 6 in]
              n144 = call "Register Event.vi"("error in (no error)"=w411, "Message"=w410, "Module ID"=w404) -> ("error out"=w408:errorcluster)  [unwired: 8 in]
              n145 = call "setSysTopics.vi"("error in (no error)"=w408, "MQTTclient in"=w409) -> ("error out"=w406:errorcluster, "List of topics"=w401:string, "MQTTclient out"=w407:refnum<class "MQTTclient.lvclass">)  [unwired: 7 in]
              n146 = Format Into String(format string="%s\nSys topic(s): %s", w400, w401) -> (resulting string=w403:string)  [unwired: 2 in, 1 out]
              n147 = in-place-cluster #2("MQTTclient"=w407) -> (w394:T2)
              n148 = call "Status Updated.vi"("error in (no error)"=w406, "Status"=w403, "Module ID"=w404) -> ("error out"=w405:errorcluster)  [unwired: 8 in]
            }
          }
          frame "disconnect" {
            n149 = Variant To Data(error in=w420, type=T6 {"Module ID"=-1, "Boolean"=FALSE} ("disconnect Argument"), Variant=w419) -> (error out=w414:errorcluster)  [unwired: 1 out]
            n150 = in-place {
              in-place-border: w414 -> [w423]
              in-place-border: [w422] -> w415
              n151 = in-place-cluster #3(w417) -> ("MQTTclient"=w424:refnum<class "MQTTclient.lvclass">)
              n152 = call-dynamic "disconnect.vi"("error in (no error)"=w423, "MQTTclient in"=w424) -> ("error out"=w422:errorcluster, "MQTTclient out"=w421:refnum<class "MQTTclient.lvclass">)  [unwired: 8 in]
              n153 = in-place-cluster #3("MQTTclient"=w421) -> (w416:T2)
            }
          }
          frame "Subscrie" {
            n154 = Variant To Data(error in=w434, type=T7 {"Module ID"=-1, "Topic"="", "Alias"=""} ("Subscrie Argument"), Variant=w433) -> (data=w431:T7, error out=w430:errorcluster)
            n155 = Unbundle By Name(w431) -> ("Alias"=w425:string, "Topic"=w428:string)
            n156 = in-place {
              in-place-border: w430 -> [w443]
              in-place-border: [w439] -> w429
              in-place-border: w428 -> [w436]
              in-place-border: w425 -> [w435]
              n157 = in-place-cluster #4(w427) -> ("MQTTclient"=w442:refnum<class "MQTTclient.lvclass">, "DICT"=w438:refnum<class "DICT.lvclass">)
              n158 = call-dynamic "Subscribe.vi"("error in (no error)"=w443, "Topic"=w436, "MQTTclient in"=w442) -> ("error out"=w440:errorcluster, "MQTTclient out"=w441:refnum<class "MQTTclient.lvclass">)  [unwired: 7 in]
              n159 = call-dynamic "Add.vi"("error in (no error)"=w440, "Alias"=w435, "Topic"=w436, "DICT in"=w438) -> ("error out"=w439:errorcluster, "DICT out"=w437:refnum<class "DICT.lvclass">)  [unwired: 6 in]
              n160 = in-place-cluster #4("MQTTclient"=w441, "DICT"=w437) -> (w426:T2)
            }
          }
          frame "unsubscribe" {
            n161 = Variant To Data(error in=w452, type=T8 {"Module ID"=-1, "Topic"=""} ("unsubscribe Argument"), Variant=w451) -> (data=w449:T8, error out=w448:errorcluster)
            n162 = Unbundle By Name(w449) -> ("Topic"=w446:string)
            n163 = in-place {
              in-place-border: w448 -> [w456]
              in-place-border: [w457] -> w447
              in-place-border: w446 -> [w453]
              n164 = in-place-cluster #5(w445) -> ("MQTTclient"=w455:refnum<class "MQTTclient.lvclass">)
              n165 = call-dynamic "Subscribe.vi"("error in (no error)"=w456, "Topic"=w453, "MQTTclient in"=w455) -> ("error out"=w457:errorcluster, "MQTTclient out"=w454:refnum<class "MQTTclient.lvclass">)  [unwired: 7 in]
              n166 = in-place-cluster #5("MQTTclient"=w454) -> (w444:T2)
            }
          }
          frame "Publish" {
            # "Publish a message to a topic"
            n167 = Variant To Data(error in=w468, type=T9 {"Module ID"=-1, "Topic"="", "Payload"=""} ("Publish Argument"), Variant=w467) -> (data=w461:T9, error out=w465:errorcluster)
            n168 = Unbundle By Name(w461) -> ("Topic"=w459:string, "Payload"=w460:string)
            n169 = case shown="\"\"" w459 {
              tunnel: w465 -> [w470 w480]
              tunnel: [w472 w479] -> w464
              tunnel: w463 -> [w474 w478]
              tunnel: [w474 w477] -> w462
              tunnel: w459 -> [_ w476]
              tunnel: w460 -> [_ w475]
              tunnel: w458 -> [w471 _]
              frame "" {
                n170 = property class="Mod Admin"(reference=w471) -> ("Accessors:Module ID"=w473:i32)  [unwired: 1 in, 2 out]
                n171 = call "Status Updated.vi"("error in (no error)"=w470, "Status"="Cannot publish on empty topic" ("format string"), "Module ID"=w473) -> ("error out"=w472:errorcluster)  [unwired: 8 in]
              }
              frame Default {
                n172 = in-place {
                  in-place-border: w480 -> [w484]
                  in-place-border: [w483] -> w479
                  in-place-border: w476 -> [w482]
                  in-place-border: w475 -> [w481]
                  n173 = in-place-cluster #6(w478) -> ("MQTTclient"=w486:refnum<class "MQTTclient.lvclass">)
                  n174 = call-dynamic "Publish.vi"("error in (no error)"=w484, "Payload"=w481, "Topic"=w482, "MQTTclient in"=w486) -> ("error out"=w483:errorcluster, "MQTTclient out"=w485:refnum<class "MQTTclient.lvclass">)  [unwired: 6 in]
                  n175 = in-place-cluster #6("MQTTclient"=w485) -> (w477:T2)
                }
              }
            }
          }
          frame "broadcastTopic" {
            # "broadcasts the message received by MQTT client"
            n176 = Variant To Data(error in=w503, type=T10 {"Module ID"=-1, "Topic"="", "Message"=""} ("broadcastTopic Argument"), Variant=w502) -> (data=w500:T10, error out=w497:errorcluster)
            n177 = Unbundle By Name(w494) -> ("MQTTclient"=w495:refnum<class "MQTTclient.lvclass">)
            n178 = Unbundle By Name(w500) -> ("Module ID"=w498:i32, "Topic"=w491:string, "Message"=w490:string)
            n179 = call-dynamic "processSysSubscription.vi"("error in (no error)"=w497, "Message"=w490, "Topic"=w491, "MQTTclient in"=w495) -> ("error out"=w496:errorcluster, "Message"=w489:string, "Topic"=w488:string, "MQTTclient out"=w492:refnum<class "MQTTclient.lvclass">, "Send?"=w487:bool)  [unwired: 3 in]
            n180 = Bundle By Name(cluster=w494, "MQTTclient"=w492) -> (w493:T2)
            n181 = case shown="False" w487 {
              tunnel: [w508 w514] -> w499
              tunnel: w498 -> [w504 w513]
              tunnel: w496 -> [w509 w512]
              tunnel: w489 -> [w506 w511]
              tunnel: w488 -> [w507 w510]
              frame False {
                n182 = call "Publish.vi"("error in (no error)"=w509, "Payload"=w506, "Topic"=w507, "Module ID"=w504) -> ("error out"=w508:errorcluster)  [unwired: 7 in]
                n183 = call "Status Updated.vi"("Status"="Sys Topic pinged" ("format string"), "Module ID"=w504) -> ()  [unwired: 9 in, 1 out]
              }
              frame True {
                n184 = call "Message.vi"("error in (no error)"=w512, "Message"=w511, "Topic"=w510, "Module ID"=w513) -> ("error out"=w514:errorcluster)  [unwired: 7 in]
              }
            }
          }
          frame "PublishByAlias" {
            n185 = Variant To Data(error in=w525, type=T11 {"Module ID"=-1, "Alias"="", "Payload"=""} ("PublishByAlias Argument"), Variant=w524) -> (data=w522:T11, error out=w521:errorcluster)
            n186 = Unbundle By Name(w522) -> ("Payload"=w519:string, "Alias"=w518:string)
            n187 = in-place {
              in-place-border: w521 -> [w533]
              in-place-border: [w535] -> w520
              in-place-border: w519 -> [w534]
              in-place-border: w518 -> [w528]
              in-place-border: w515 -> [w526]
              n188 = in-place-cluster #7(w517) -> ("MQTTclient"=w537:refnum<class "MQTTclient.lvclass">, "DICT"=w529:refnum<class "DICT.lvclass">)
              n189 = call-dynamic "getTopic.vi"("error in (no error)"=w533, "Alias"=w528, "DICT in"=w529) -> ("error out"=w532:errorcluster, "TopicFound"=w527:bool, "Topic"=w531:string, "DICT out"=w530:refnum<class "DICT.lvclass">)  [unwired: 5 in]
              n190 = case shown="False" w527 {
                tunnel: w537 -> [w543 w549]
                tunnel: [w543 w548] -> w536
                tunnel: [w539 w547] -> w535
                tunnel: w534 -> [_ w546]
                tunnel: w532 -> [w540 w545]
                tunnel: w531 -> [_ w544]
                tunnel: w526 -> [w538 _]
                frame False {
                  n191 = property class="Mod Admin"(reference=w538) -> ("Accessors:Module ID"=w542:i32)  [unwired: 1 in, 2 out]
                  n192 = call "Status Updated.vi"("error in (no error)"=w540, "Status"="Alias not found" ("format string"), "Module ID"=w542) -> ("error out"=w539:errorcluster)  [unwired: 8 in]
                }
                frame True {
                  n193 = call-dynamic "Publish.vi"("error in (no error)"=w545, "Payload"=w546, "Topic"=w544, "MQTTclient in"=w549) -> ("error out"=w547:errorcluster, "MQTTclient out"=w548:refnum<class "MQTTclient.lvclass">)  [unwired: 6 in]
                }
              }
              n194 = in-place-cluster #7("MQTTclient"=w536, "DICT"=w530) -> (w516:T2)
            }
          }
          frame "addTopicAlias" {
            n195 = property class="Mod Admin"(reference=w552) -> ("Accessors:Module ID"=w551:i32)  [unwired: 1 in, 2 out]
            n196 = Variant To Data(error in=w566, type=T12 {"Module ID"=-1, "Topic"="", "Alias"=""} ("addTopicAlias Argument"), Variant=w565) -> (data=w563:T12, error out=w562:errorcluster)
            n197 = Unbundle By Name(w563) -> ("Topic"=w559:string, "Alias"=w558:string)
            n198 = Empty String/Path?(string/path=w558) -> (empty?=w557:bool)
            n199 = Empty String/Path?(string/path=w559) -> (empty?=w556:bool)
            n200 = Or(x=w557, y=w556) -> (x .or. y?=w555:bool)
            n201 = case shown="False" w555 {
              tunnel: w562 -> [w573 w586]
              tunnel: w561 -> [w572 w587]
              tunnel: [w571 w587] -> w560
              tunnel: [w570 w586] -> w554
              tunnel: w559 -> [w569 w583]
              tunnel: w558 -> [w568 w584]
              tunnel: [w567 w582] -> w550
              frame False {
                n202 = in-place {
                  in-place-border: w573 -> [w581]
                  in-place-border: [w580] -> w570
                  in-place-border: w569 -> [w575]
                  in-place-border: w568 -> [w576]
                  in-place-border: [w574] -> w567
                  n203 = in-place-cluster #8(w572) -> ("DICT"=w579:refnum<class "DICT.lvclass">)
                  n204 = call-dynamic "Add.vi"("error in (no error)"=w581, "Alias"=w576, "Topic"=w575, "DICT in"=w579) -> ("error out"=w580:errorcluster, "DICT out"=w578:refnum<class "DICT.lvclass">)  [unwired: 6 in]
                  n205 = Format Into String(format string="Alias <<%s>>: <<%s>>\n created!", w576, w575) -> (resulting string=w574:string)  [unwired: 2 in, 1 out]
                  n206 = in-place-cluster #8("DICT"=w578) -> (w571:T2)
                }
              }
              frame True {
                n207 = Format Into String(format string="Alias <<%s>>: <<%s>>\nnot created!", w584, w583) -> (resulting string=w582:string)  [unwired: 2 in, 1 out]
              }
            }
            n208 = call "Status Updated.vi"("error in (no error)"=w554, "Status"=w550, "Module ID"=w551) -> ("error out"=w553:errorcluster)  [unwired: 8 in]
          }
          frame "---Copy This Frame---" {
            # "Duplicate this frame when creating new messages.  Change this comment in the duplicated frame to describe this message."
            n209 = Merge Errors(w590) -> (w588:errorcluster)
          }
          frame "--- Exit and Error Handling---" {
            # "Separator - the following cases handle errors and exit messages."
            n210 = Merge Errors(w593) -> (w591:errorcluster)
          }
          frame "Error" {
            # "#CodeRecommended - If you ever change the name of this \"Error\" message, you'll need to update the name in the Check Loop Error.vi as well."
            # "#CodeRecommended - If the module is running in standalone mode (External Launch = FALSE), this code will pop up an error dialog and call the 'Exit' message if an error occurs. Add more fine-grained error handling here."
            # "Error - Check the error message data and respond accordingly. This message is sent by the \"Error Handler\" VIs at the end of each loop in this application."
            n211 = property class="Mod Admin"(reference=w599) -> ("Accessors:External Launch"=w596:bool, "Accessors:Module ID"=w598:i32)  [unwired: 1 in, 2 out]
            n212 = Variant To Data(error in=w604, type=errorcluster {"status"=FALSE, "code"=0, "source"=""} ("error constant"), Variant=w602) -> (data=w605:errorcluster, error out=w600:errorcluster)
            n213 = call "Error Reported.vi"("Error"=w605, "Module ID"=w598) -> ()  [unwired: 9 in, 1 out]
            n214 = case shown="False" w596 {
              tunnel: [w610 _] -> w597
              tunnel: w595 -> [w609 _]
              tunnel: w605 -> [w606 _]
              frame False {
                # "If the module is running standalone, then pop up an error dialog and call the \"Exit\" message."
                n215 = call <vilib>:"Simple Error Handler.vi"("error in (no error)"=w606) -> ()  [unwired: 4 in, 5 out]
                n216 = call-poly <vilib>:"Delacor_lib_QMH_Enqueue Message (poly).vi"("Priority Message? (F)"=TRUE, "Message"="Exit", "Message Queue in"=w609) -> ("error out"=w610:errorcluster)  [unwired: 7 in, 1 out]
              }
              frame True {
                # "If the module was launched externally, calling the Error Reported broadcast VI is the only action performed by the \"Error\" message. The module's caller can then process the error appropriately."
              }
            }
            n217 = Merge Errors(w600, w597) -> (w594:errorcluster)
            n218 = local write "error out"(w594) -> ()
          }
          frame "Simulate MHL Error" {
            # "Simulate an error occurring at the MHL"
            n219 = property class="Mod Admin"(reference=w612) -> ("Accessors:Module ID"=w613:i32)  [unwired: 1 in, 2 out]
            n220 = call "Module Name--constant.vi"("Module ID"=w613) -> ("Module Name"=w611:string)  [unwired: 10 in]
            n221 = xnode "Error Ring"("parameter 0"=w611) -> ("error out"=w614:errorcluster)
            n222 = Merge Errors(w617, w614) -> (w615:errorcluster)
          }
          frame "Confirm Quit" {
            # "#CodeNeeded - If you want to provide an \"Are you sure\" dialog (or some other notification) before the application exits, place that code here. This message is typically sent from a Panel Close? event."
            # "Confirm Quit - Message that can confirm whether or not the user wants to exit this instance."
            n223 = call-poly <vilib>:"Delacor_lib_QMH_Enqueue Message (poly).vi"("Priority Message? (F)"=TRUE, "error in (no error)"=w627, "Message"="Exit", "Message Queue in"=w628) -> ("error out"=w630:errorcluster)  [unwired: 6 in, 1 out]
            n224 = Merge Errors(w630) -> (w626:errorcluster)
          }
          frame "Exit" {
            w644 = 91  # 91: not all Exit messages will have an argument
            w648 = TRUE  # Stop the VI
            # "Release the message queue reference"
            # "Exit - Exit the application."
            n225 = Variant To Data(error in=w651, type=T3 {"Origin"="", "Module ID"=-1, "Exit via Stop Module Req?"=FALSE, "Wait for Module to stop?"=FALSE} ("Stop Argument"), Variant=w642) -> (data=w639:T3, error out=w643:errorcluster)
            n226 = call <vilib>:"Clear Errors.vi"("error in (no error)"=w643, "specific error code to clear (0: all)"=w644) -> ("error out"=w650:errorcluster)  [unwired: 4 in, 1 out]
            n227 = Unbundle By Name(w633) -> ("MQTTclient"=w636:refnum<class "MQTTclient.lvclass">)
            n228 = Unbundle By Name(w633) -> ("DICT"=w634:refnum<class "DICT.lvclass">)
            n229 = control-ref of="This VI"() -> (w637:refnum<vi>)
            n230 = call-dynamic "Delacor_lib_QMH_Release Message Queue.vi"("error in (no error)"=w650, "Message Queue"=w649) -> ("error out"=w647:errorcluster)  [unwired: 9 in]
            n231 = call "Handle Exit.vi"("Stop Argument"=w639, "Module Admin in"=w638, "VI reference"=w637) -> ("error out"=w645:errorcluster, "Wait for Stop?"=w640:bool)  [unwired: 7 in]
            n232 = call-dynamic "clear.vi"("DICT in"=w634) -> ("error out"=w632:errorcluster)  [unwired: 9 in, 1 out]
            n233 = call-dynamic "disconnect.vi"("MQTTclient in"=w636) -> ("error out"=w635:errorcluster)  [unwired: 9 in, 1 out]
            n234 = call <vilib>:"Clear Errors.vi"("error in (no error)"=w632) -> ()  [unwired: 5 in, 2 out]
            n235 = call <vilib>:"Clear Errors.vi"("error in (no error)"=w635) -> ()  [unwired: 5 in, 2 out]
            n236 = Merge Errors(w645, w647) -> (w646:errorcluster)
          }
          frame Default {
            # "'Default' case only runs if there is a message that isn't defined in any of the other cases.  Output a programming error."
            n237 = property class="Mod Admin"(reference=w653) -> ("Accessors:Module ID"=w652:i32)  [unwired: 1 in, 2 out]
            n238 = call "Module Name--constant.vi"("Module ID"=w652) -> ("Module Name"=w654:string)  [unwired: 10 in]
            n239 = xnode "Error Ring"("parameter 0"=w655, "parameter 1"=w654) -> ("error out"=w656:errorcluster)
          }
        }
        n240 = call-dynamic "Delacor_lib_QMH_Error Handler - Message Handling Loop.vi"("error in (no error)"=w305, "Message Queue in"=w296) -> ("dup error in"=w295:errorcluster)  [unwired: 8 in, 1 out]
      }
    }
    frame Error {
      n241 = call "Synchronize Caller Events.vi"("Module Admin"=w668) -> ("Module Admin out"=w667:refnum<class "Delacor_lib_QMH_Cloneable Module Admin.lvclass">)  [unwired: 9 in, 1 out]
      n242 = property class="Mod Admin"(reference=w667) -> ("Accessors:Module ID"=w666:i32)  [unwired: 1 in, 2 out]
      n243 = call "Module Name--constant.vi"("Module ID"=w666) -> ("Module Name"=w671:string)  [unwired: 10 in]
      n244 = call "Remove.vi"("Module ID"=w666) -> ()  [unwired: 9 in, 2 out]
      n245 = Format Into String(format string="An error occurred during initialization. %s is no longer running.", w671) -> (resulting string=w669:string)  [unwired: 2 in, 1 out]
      n246 = call "Error Reported.vi"("Additional Information"=w669, "Error"=w672, "Module ID"=w666) -> ()  [unwired: 8 in, 1 out]
    }
  }
  n247 = Merge Errors(w16, w15) -> (w17:errorcluster)
  n248 = call "Close Module.vi"("error in (no error)"=w17, "Wait for stop?"=w5, "Module Admin in"=w7) -> ("error out"=w9:errorcluster, "External Launch"=w3:bool, "Module Admin out"=w6:refnum<class "Delacor_lib_QMH_Cloneable Module Admin.lvclass">)  [unwired: 6 in]
  n249 = Unregister For Events(event registration refnum=w13, error in=w9) -> (error out=w4:errorcluster)
  "error out" <- w4
  n250 = local write "Module Admin"(w6) -> ()
  n251 = case "External Launch?" shown="True" w3 {
    tunnel: w4 -> [_ w674]
    frame False {
    }
    frame True {
      n252 = case shown="No Error" w674 {
        frame No Error {
          n253 = invoke class="VI" method="FP.Close"() -> ()  [unwired: 3 in, 3 out]
        }
        frame Error {
          n254 = invoke class="VI" method="FP.Open"("Activate"=TRUE ("Activate?")) -> ()  [unwired: 4 in, 5 out]
        }
      }
    }
  }
